vi "Read Serial Number.vi"(7 "Unit ID (A)":string="A", 8 "error in":errorcluster, 11 "VISA Session In":refnum<visa-resource-name>="Alicat") -> (0 "error out":errorcluster, 2 "Serial Number":i32, 3 "VISA Session Out":refnum<visa-resource-name>)   [LabVIEW 2015]
doc: "Returns the serial number of the queried Alicat device."
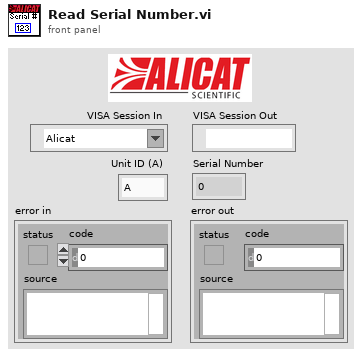
[diagram p1: front panel]
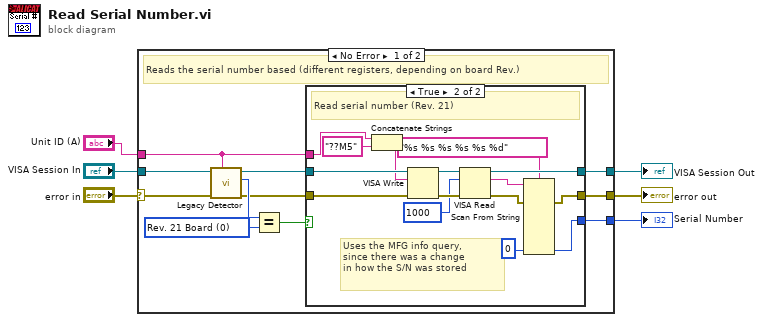
[diagram p0: block diagram]
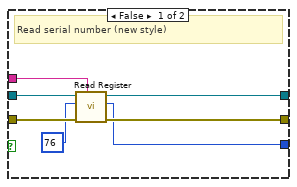
[diagram p2: hidden frame]
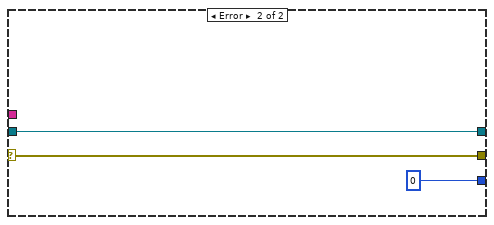
[diagram p3: hidden frame]
diagram:
  n1 = case shown="No Error" "error in" {
    selector: "error in" -> [w7 w41]
    tunnel: [w14 w42] -> w6
    tunnel: [w13 w41] -> w5
    tunnel: "VISA Session In" -> [w10 w42]
    tunnel: "Unit ID (A)" -> [w9 _]
    tunnel: [w8 0 ("Register Value (I32)")] -> w2
    frame No Error {
      w16 = u8 0 items=["Rev. 21 Board", "Rev. 22 Board", "Rev. 23 Board"] ("Legacy Status")
      # "Reads the serial number based (different registers, depending on board Rev.)"
      n2 = call "Legacy Detector.vi"("Unit ID (A)"=w9, "error in"=w7, "VISA Session In"=w10) -> ("error out"=w12:errorcluster, "Legacy Status"=w15:u8, "VISA Session Out"=w11:refnum<visa-resource-name>)  [unwired: 6 in]
      n3 = Equal?(x=w15, y=w16) -> (x = y?=w17:bool)
      n4 = case shown="True" w17 {
        tunnel: w12 -> [w23 w36]
        tunnel: [w24 w28] -> w13
        tunnel: [w22 w31] -> w14
        tunnel: w11 -> [w21 w35]
        tunnel: w9 -> [w18 w34]
        tunnel: [w20 w25] -> w8
        frame False {
          # "Read serial number (new style)"
          n5 = call "Read Register.vi"("Unit ID (A)"=w18, "error in"=w23, "Register address"=u16 76, "VISA Session In"=w21) -> ("error out"=w24:errorcluster, "Register Value (I32)"=w20:i32, "VISA Session Out"=w22:refnum<visa-resource-name>)  [unwired: 5 in]
        }
        frame True {
          # "Uses the MFG info query,\nsince there was a change\nin how the S/N was stored"
          # "Read serial number (Rev. 21)"
          n6 = Concatenate Strings(w34, "??M5" ("string")) -> (w32:string)
          n7 = VISA Write(VISA resource name=w35, write buffer=w32, error in (no error)=w36) -> (VISA resource name out=w38:refnum<visa-resource-name>, error out=w39:errorcluster)  [unwired: 1 out]
          n8 = VISA Read(VISA resource name=w38, byte count=u32 1000, error in (no error)=w39) -> (VISA resource name out=w31:refnum<visa-resource-name>, read buffer=w30:string, error out=w27:errorcluster)  [unwired: 1 out]
          n9 = Scan From String(format string="%s %s %s %s %s %d", input string=w30, error in=w27, default 6=0 ("default value 5")) -> (error out=w28:errorcluster, output 6=w25:i32)  [unwired: 11 in, 2 out]
        }
      }
    }
    frame Error {
    }
  }
  "error out" <- w5
  "VISA Session Out" <- w6
  "Serial Number" <- w2
